vi "RT Main.vi"() -> ()   [LabVIEW 2013]
doc: "This template is for the Queued Message Handler design pattern.\n\nThe Event Handling Loop generates messages based on user interface actions.\n\nThe Message Handling Loop processes messages generated by the Event Handling Loop, or by other messages. The messages are string values, so new messages can be added easily to the Message Cases case structure in the Message Handling Loop. Each message cluster can also provide an optional value for Message Data, which is a variant that can be converted to whatever message-specific data is required."
uses:
  controls/Custom Controller Inputs.ctl
  <vilib>/userdefined/High Color/nirio_resource_hc.ctl
  controls/FPGA State.ctl
  controls/Raw Values.ctl
  controls/Control Configuration.ctl
  Globals/Global - All RT Loop Stop.vi
  Globals/Global - Configuration Options.vi
  <vilib>/rvi/errors/niLvFpgaAdjustHostInterfaceError.vi
  Globals/Global - RT Stream Connections.vi
  <vilib>/FPGAPlugInAG/cRIO-9075/niLvFpga_Close_cRIO-9075.vi
  <vilib>/rvi/interface/nirviReadWriteControl/nirviReadWriteControl.xnode
  controls/FPGA VI Reference.ctl
  FPGA Bitfiles/crio-FPGA-contro_FPGATarget_FPGAMain_4HKUk4gb9wY.lvbitx
  <vilib>/rvi/interface/nirviCloseFPGA/nirviCloseFPGA.xnode
  support/Message Queue/Message Queue.lvlib
  NiFpgaLv.dll
  <vilib>/nisyscfg/nisyscfg.lvlib
panel:
  in  "resource name":T1
  in  "Custom Controller Inputs":T2
  out "Data":T3 {"Other Controller Gains"."Position Control Kp" format="%.11g"; "Other Controller Gains"."Virtual Spring Constant (N/m)" format="%.8g"; "Other Controller Gains"."Offset weight (N)" format="%.11g"; "Other Controller Gains"."Fthresh (N)" format="%.13g"; "Other Controller Gains"."Var2" format="%.13g"}
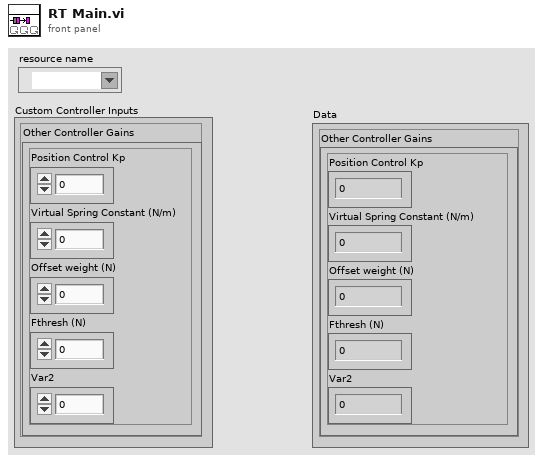
[diagram p1: front panel]
types:
  T1 = typedef "nirio_resource_hc.ctl" = tag
  T2 = typedef "Custom Controller Inputs.ctl" = cluster{"Other Controller Gains":cluster{"Position Control Kp":fxp<+/-,16,8>, "Virtual Spring Constant (N/m)":fxp<+,16,12>, "Offset weight (N)":fxp<+/-,16,8>, "Fthresh (N)":fxp<+/-,16,5>, "Var2":fxp<+/-,16,5>}}
  T3 = cluster{"Other Controller Gains":cluster{"Position Control Kp":fxp<+/-,16,8>, "Virtual Spring Constant (N/m)":fxp<+,16,12>, "Offset weight (N)":fxp<+/-,16,8>, "Fthresh (N)":fxp<+/-,16,5>, "Var2":fxp<+/-,16,5>}}
  T4 = typedef "FPGA VI Reference.ctl" = refnum<k20>
  T5 = typedef "FPGA State.ctl" = enum16{"Safe State", "Manual", "Control (PID)"}
  T6 = typedef "Raw Values.ctl" = cluster{"Channel 0":fxp<+/-,20,7>, "Channel 1":fxp<+/-,20,7>, "Channel 2":fxp<+/-,20,7>, "Channel 3":fxp<+/-,20,14>}
  T7 = typedef "Control Configuration.ctl" = cluster{"PID Gains":cluster{"proportional gain (Kc)":fxp<+/-,16,8>, "integral gain (Kc*Ts/Ti)":fxp<+/-,16,8>, "derivative gain (Kc*Td/Ts)":fxp<+/-,16,8>}, "Output Range":cluster{"output high":fxp<+/-,16,7>, "output low":fxp<+/-,16,7>}}
  T8 = typedef "All FPGA Configuration Values.ctl" = cluster{"FPGA State":T5, "Manual Values":T6, "Setpoints":T6, "Control Configurations":T7[]}
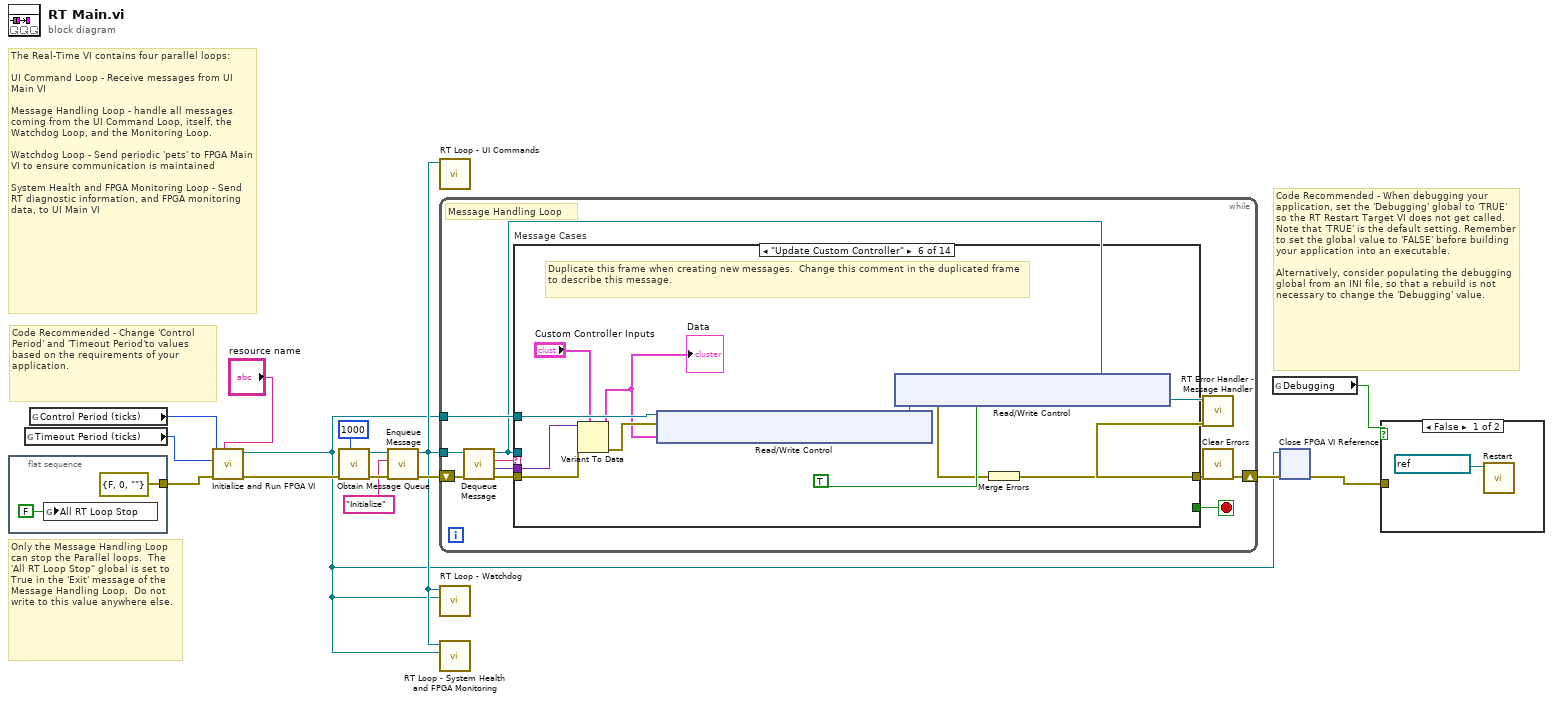
[diagram p0: block diagram]
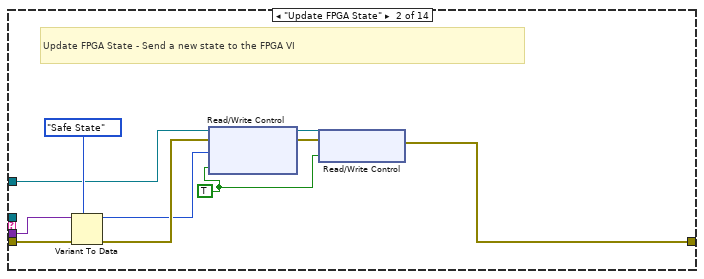
[diagram p4: hidden frame]
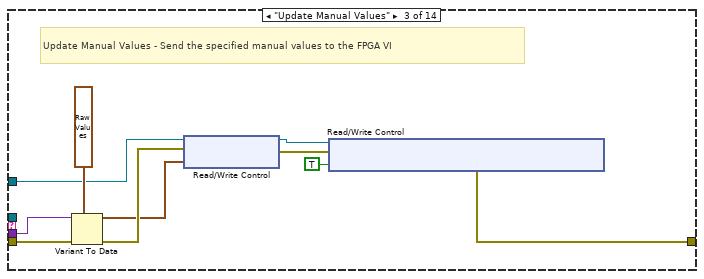
[diagram p5: hidden frame]
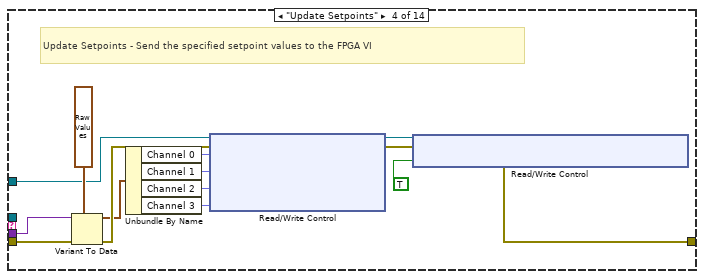
[diagram p6: hidden frame]
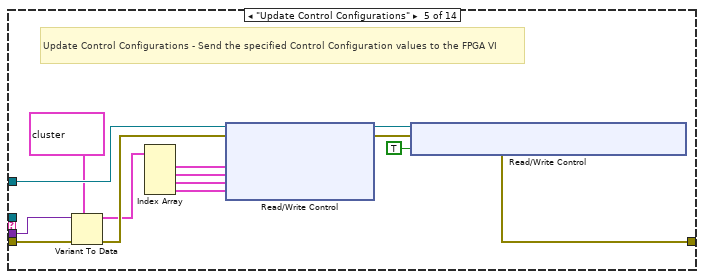
[diagram p7: hidden frame]
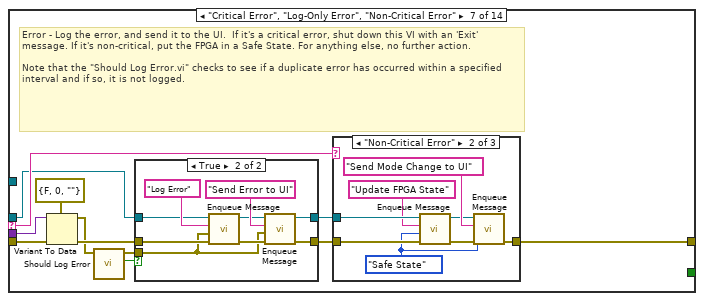
[diagram p8: hidden frame]
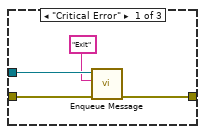
[diagram p10: hidden frame]
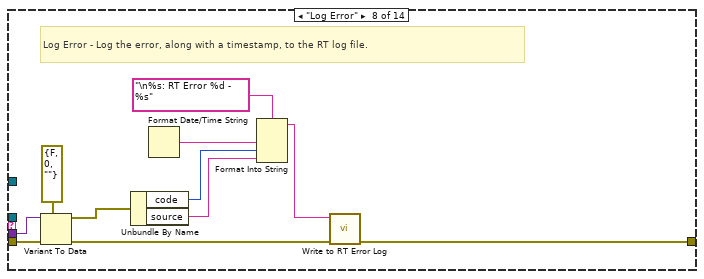
[diagram p12: hidden frame]
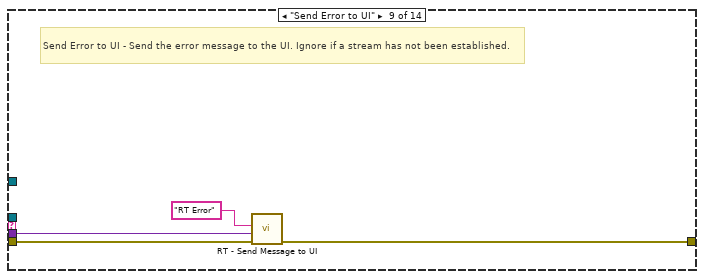
[diagram p13: hidden frame]
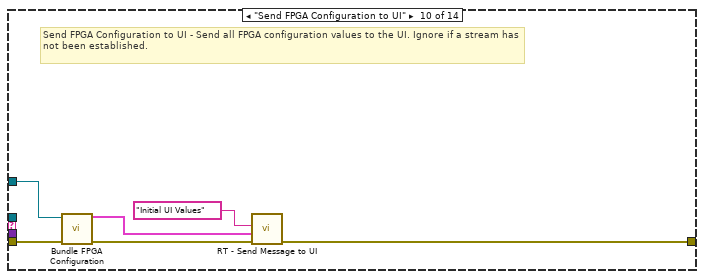
[diagram p14: hidden frame]
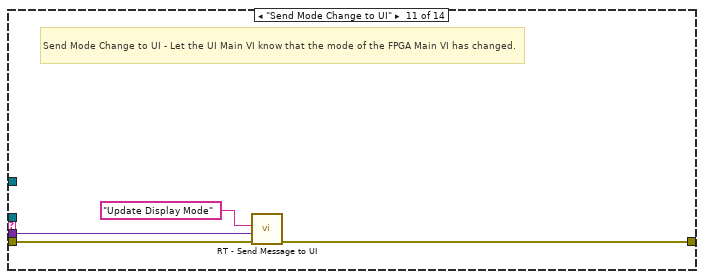
[diagram p15: hidden frame]
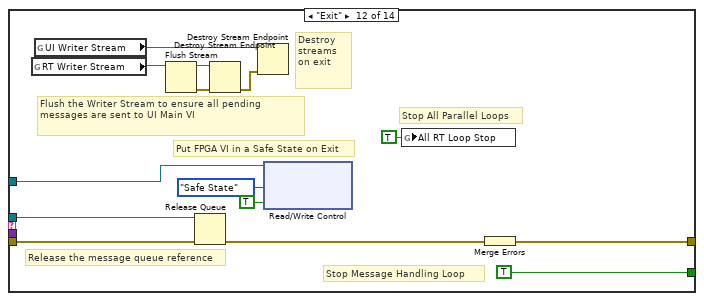
[diagram p16: hidden frame]
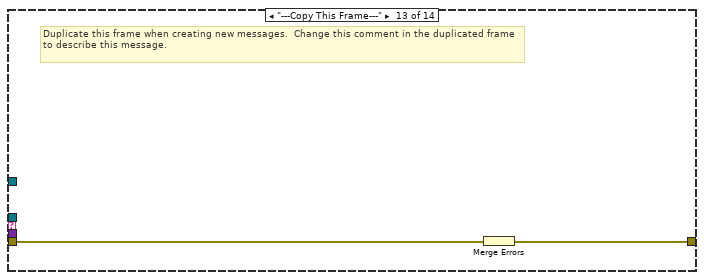
[diagram p17: hidden frame]
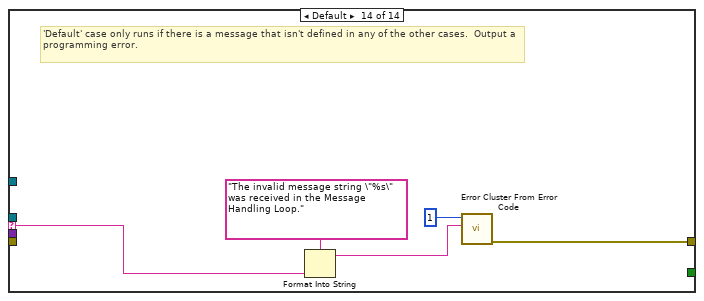
[diagram p18: hidden frame]
diagram:
  # "Code Recommended - When debugging your application, set the 'Debugging' global to 'TRUE' so the RT Restart Target VI does not get called.  Note that 'TRUE' is the default setting. Remember to set the global value to 'FALSE' before building your application into an executable.\n\nAlternatively, consider populating the debugging global from an INI file, so that a rebuild is not necessary to change the 'Debugging' value."
  # "Code Recommended - Change 'Control Period' and 'Timeout Period'to values based on the requirements of your application."
  # "The Real-Time VI contains four parallel loops:\n\nUI Command Loop - Receive messages from UI Main VI\n\nMessage Handling Loop - handle all messages coming from the UI Command Loop, itself, the Watchdog Loop, and the Monitoring Loop.\n\nWatchdog Loop - Send periodic 'pets' to FPGA Main VI to ensure communication is maintained\n\nSystem Health and FPGA Monitoring Loop - Send RT diagnostic information, and FPGA monitoring data, to UI Main VI"
  # "Only the Message Handling Loop can stop the Parallel loops.  The 'All RT Loop Stop\" global is set to True in the 'Exit' message of the Message Handling Loop.  Do not write to this value anywhere else."
  n1 = flat-sequence {
    tunnel: [errorcluster {"status"=FALSE, "code"=0, "source"=""} ("error constant")] -> w5
    frame #0 {
      n2 = global write "Global - All RT Loop Stop.vi" "All RT Loop Stop"(FALSE) -> ()
    }
  }
  n3 = global read "Global - Configuration Options.vi" "Timeout Period (ticks)"() -> (w3:u64)
  n4 = global read "Global - Configuration Options.vi" "Control Period (ticks)"() -> (w4:u32)
  n5 = call "Initialize and Run FPGA VI.vi"("resource name"="resource name", "error in (no error)"=w5, "Timeout Period (ticks)"=w3, "Control Period (ticks)"=w4) -> ("error out"=w6:errorcluster, "FPGA VI Reference Out"=w2:T4)  [unwired: 6 in]
  n6 = call "Obtain Message Queue.vi"("max queue size (-1, unlimited)"=1000, "error in (no error)"=w6) -> ("error out"=w15:errorcluster, "Message Queue"=w14:refnum<queue>)  [unwired: 8 in]
  n7 = call "Enqueue Message.vi"("error in (no error)"=w15, "Message"="Initialize", "Message Queue"=w14) -> ("error out"=w12:errorcluster, "dup Message Queue"=w11:refnum<queue>)  [unwired: 7 in]
  n8 = call "RT Loop - UI Commands.vi"("Message Queue"=w11) -> ()  [unwired: 11 in]
  n9 = while {
    tunnel: w11 -> [w22]
    shift-right: [w19] -> w10
    shift-left: w12 -> [w26]
    tunnel: w2 -> [w21]
    stop <- w27 stop-if-true
    # "Message Handling Loop"
    n10 = call "Dequeue Message.vi"("error in (no error)"=w26, "Message Queue"=w22) -> ("error out"=w25:errorcluster, "Message Data"=w23:variant, "Message"=w24:string, "dup Message Queue"=w20:refnum<queue>)  [unwired: 6 in]
    n11 = case "Message Cases" shown="\"Update Custom Controller\"" w24 {
      selector: w24 -> [_ _ _ _ _ _ w97 _ _ _ _ _ _ w168]
      tunnel: w20 -> [_ _ _ _ _ _ w91 _ _ _ _ w162 _ _]
      tunnel: w25 -> [w28 w38 w48 w62 w76 w86 w95 w134 w138 w144 w148 w158 w164 _]
      tunnel: [w28 w30 w39 w49 w63 w87 w96 w125 w135 w139 w147 w159 w163 w166] -> w18
      tunnel: [_ _ _ _ _ _ _ _ _ _ _ TRUE _ _] -> w27
      tunnel: w23 -> [_ w37 w47 w61 w75 w85 w94 w133 w137 _ w146 _ _ _]
      tunnel: w21 -> [_ w34 w44 w58 w73 w84 _ _ _ w143 _ w154 _ _]
      frame "Initialize" {
        # "Initialize - Currently a no-op for the RT Main VI"
      }
      frame "Update FPGA State" {
        w29 = TRUE ("Change State")
        # "Update FPGA State - Send a new state to the FPGA VI"
        n12 = Variant To Data(error in=w38, type=FPGA_State."Safe State" ("FPGA State"), Variant=w37) -> (data=w33:T5, error out=w35:errorcluster)
        n13 = xnode "Read/Write Control"("FPGA VI Reference In"=w34, "error in"=w35, "New State"=w33, "Change State"=w29) -> ("FPGA VI Reference Out"=w32:T4, "error out"=w31:errorcluster)
        n14 = xnode "Read/Write Control"("FPGA VI Reference In"=w32, "error in"=w31, "Disable Drive"=w29) -> ("error out"=w30:errorcluster)  [unwired: 1 out]
      }
      frame "Update Manual Values" {
        # "Update Manual Values - Send the specified manual values to the FPGA VI"
        n15 = Variant To Data(error in=w48, type=T6 {"Channel 0"=0.0, "Channel 1"=0.0, "Channel 2"=0.0, "Channel 3"=0.0} ("Raw Values"), Variant=w47) -> (data=w43:T6, error out=w45:errorcluster)
        n16 = xnode "Read/Write Control"("FPGA VI Reference In"=w44, "error in"=w45, "Manual Values"=w43) -> ("FPGA VI Reference Out"=w42:T4, "error out"=w41:errorcluster)
        n17 = xnode "Read/Write Control"("FPGA VI Reference In"=w42, "error in"=w41, "Enable Drive"=TRUE) -> ("error out"=w39:errorcluster)  [unwired: 1 out]
      }
      frame "Update Setpoints" {
        # "Update Setpoints - Send the specified setpoint values to the FPGA VI"
        n18 = Variant To Data(error in=w62, type=T6 {"Channel 0"=0.0, "Channel 1"=0.0, "Channel 2"=0.0, "Channel 3"=0.0} ("Raw Values"), Variant=w61) -> (data=w57:T6, error out=w59:errorcluster)
        n19 = Unbundle By Name(w57) -> ("Channel 0"=w56:fxp<+/-,20,7>, "Channel 1"=w53:fxp<+/-,20,7>, "Channel 2"=w55:fxp<+/-,20,7>, "Channel 3"=w54:fxp<+/-,20,14>)
        n20 = xnode "Read/Write Control"("FPGA VI Reference In"=w58, "error in"=w59, "Channel 0 Setpoint (Force)"=w56, "Channel 1 Setpoint  (Position)"=w53, "Channel 2 Setpoint"=w55, "Channel 3 Setpoint"=w54) -> ("FPGA VI Reference Out"=w50:T4, "error out"=w51:errorcluster)
        n21 = xnode "Read/Write Control"("FPGA VI Reference In"=w50, "error in"=w51, "Enable Drive"=TRUE) -> ("error out"=w49:errorcluster)  [unwired: 1 out]
      }
      frame "Update Control Configurations" {
        # "Update Control Configurations - Send the specified Control Configuration values to the FPGA VI"
        n22 = Variant To Data(error in=w76, type=T7[] [{"PID Gains"={"proportional gain (Kc)"=0.0, "integral gain (Kc*Ts/Ti)"=0.0, "derivative gain (Kc*Td/Ts)"=0.0}, "Output Range"={"output high"=0.0, "output low"=0.0}}], Variant=w75) -> (data=w71:T7[], error out=w74:errorcluster)
        n23 = Index Array(array=w71) -> (element #1=w70:T7, element #2=w69:T7, element #3=w68:T7, element #4=w67:T7)  [unwired: 4 in]
        n24 = xnode "Read/Write Control"("FPGA VI Reference In"=w73, "error in"=w74, "Channel 0 Configuration"=w70, "Channel 1 Configuration"=w69, "Channel 2 Configuration"=w68, "Channel 3 Configuration"=w67) -> ("FPGA VI Reference Out"=w65:T4, "error out"=w64:errorcluster)
        n25 = xnode "Read/Write Control"("FPGA VI Reference In"=w65, "error in"=w64, "Enable Drive"=TRUE) -> ("error out"=w63:errorcluster)  [unwired: 1 out]
      }
      frame "Update Custom Controller" {
        # "Duplicate this frame when creating new messages.  Change this comment in the duplicated frame to describe this message."
        n26 = Variant To Data(error in=w86, type="Custom Controller Inputs", Variant=w85) -> (data=w78:T2, error out=w83:errorcluster)
        "Data" <- w78
        n27 = xnode "Read/Write Control"("FPGA VI Reference In"=w84, "error in"=w83, "Custom Controller Inputs"=w78) -> ("FPGA VI Reference Out"=w81:T4, "error out"=w80:errorcluster)
        n28 = xnode "Read/Write Control"("FPGA VI Reference In"=w81, "error in"=w80, "Enable Drive"=TRUE) -> ("error out"=w79:errorcluster)  [unwired: 1 out]
        n29 = Merge Errors(w79) -> (w87:errorcluster)
      }
      frame "Critical Error", "Log-Only Error", "Non-Critical Error" {
        # "Error - Log the error, and send it to the UI.  If it's a critical error, shut down this VI with an 'Exit' message. If it's non-critical, put the FPGA in a Safe State. For anything else, no further action.\n\nNote that the \"Should Log Error.vi\" checks to see if a duplicate error has occurred within a specified interval and if so, it is not logged."
        n30 = Variant To Data(error in=w95, type=errorcluster {"status"=FALSE, "code"=0, "source"=""} ("error out"), Variant=w94) -> (data=w89:errorcluster, error out=w92:errorcluster)
        n31 = call "Should Log Error.vi"("error to report"=w89) -> ("Should Log Error?"=w90:bool, "dup error to report"=w88:errorcluster)  [unwired: 9 in]
        n32 = case shown="True" w90 {
          tunnel: [w101 w108] -> w99
          tunnel: [w100 w107] -> w98
          tunnel: w91 -> [w100 w106]
          tunnel: w92 -> [w101 w103]
          tunnel: w88 -> [_ w102]
          frame False {
          }
          frame True {
            n33 = call "Enqueue Message.vi"("error in (no error)"=w103, "Message Data"=w102, "Message"="Log Error", "Message Queue"=w106) -> ("error out"=w104:errorcluster, "dup Message Queue"=w105:refnum<queue>)  [unwired: 6 in]
            n34 = call "Enqueue Message.vi"("error in (no error)"=w104, "Message Data"=w102, "Message"="Send Error to UI", "Message Queue"=w105) -> ("error out"=w108:errorcluster, "dup Message Queue"=w107:refnum<queue>)  [unwired: 6 in]
          }
        }
        n35 = case shown="\"Non-Critical Error\"" w97 {
          tunnel: w99 -> [w114 w122 w123]
          tunnel: w98 -> [w112 w121 _]
          tunnel: [w113 w118 w123] -> w96
          frame "Critical Error" {
            n36 = call "Enqueue Message.vi"("error in (no error)"=w114, "Message"="Exit", "Message Queue"=w112) -> ("error out"=w113:errorcluster)  [unwired: 7 in, 1 out]
          }
          frame "Non-Critical Error" {
            w115 = FPGA_State."Safe State" ("FPGA State")
            n37 = call "Enqueue Message.vi"("error in (no error)"=w122, "Message Data"=w115, "Message"="Update FPGA State", "Message Queue"=w121) -> ("error out"=w119:errorcluster, "dup Message Queue"=w116:refnum<queue>)  [unwired: 6 in]
            n38 = call "Enqueue Message.vi"("error in (no error)"=w119, "Message Data"=w115, "Message"="Send Mode Change to UI", "Message Queue"=w116) -> ("error out"=w118:errorcluster)  [unwired: 6 in, 1 out]
          }
          frame Default {
          }
        }
      }
      frame "Log Error" {
        # "Log Error - Log the error, along with a timestamp, to the RT log file."
        n39 = Variant To Data(error in=w134, type=errorcluster {"status"=FALSE, "code"=0, "source"=""} ("error constant"), Variant=w133) -> (data=w128:errorcluster, error out=w131:errorcluster)
        n40 = Unbundle By Name(w128) -> ("code"=w127:i32, "source"=w126:string)
        n41 = Format Date/Time String() -> (date/time string=w129:string)  [unwired: 3 in]
        n42 = Format Into String(format string="\n%s: RT Error %d - %s", w129, w127, w126) -> (resulting string=w124:string)  [unwired: 2 in, 1 out]
        n43 = call "Write to RT Error Log.vi"("error in (no error)"=w131, "Log Entry"=w124) -> ("error out"=w125:errorcluster)  [unwired: 9 in]
      }
      frame "Send Error to UI" {
        # "Send Error to UI - Send the error message to the UI. Ignore if a stream has not been established."
        n44 = call "RT - Send Message to UI.vi"("error in (no error)"=w138, "Message Data"=w137, "Message"="RT Error") -> ("error out"=w135:errorcluster)  [unwired: 8 in]
      }
      frame "Send FPGA Configuration to UI" {
        # "Send FPGA Configuration to UI - Send all FPGA configuration values to the UI. Ignore if a stream has not been established."
        n45 = call "Bundle FPGA Configuration.vi"("error in (no error)"=w144, "FPGA Interface (Old)"=w143) -> ("error out"=w142:errorcluster, "All FPGA Configuration Values"=w141:T8)  [unwired: 8 in]
        n46 = call "RT - Send Message to UI.vi"("error in (no error)"=w142, "Message Data"=w141, "Message"="Initial UI Values") -> ("error out"=w139:errorcluster)  [unwired: 8 in]
      }
      frame "Send Mode Change to UI" {
        # "Send Mode Change to UI - Let the UI Main VI know that the mode of the FPGA Main VI has changed."
        n47 = call "RT - Send Message to UI.vi"("error in (no error)"=w148, "Message Data"=w146, "Message"="Update Display Mode") -> ("error out"=w147:errorcluster)  [unwired: 8 in]
      }
      frame "Exit" {
        # "Flush the Writer Stream to ensure all pending messages are sent to UI Main VI"
        # "Destroy streams on exit"
        # "Put FPGA VI in a Safe State on Exit"
        # "Stop Message Handling Loop"
        # "Stop All Parallel Loops"
        # "Release the message queue reference"
        n48 = global read "Global - RT Stream Connections.vi" "RT Writer Stream"() -> (w151:refnum<k21>)
        n49 = global read "Global - RT Stream Connections.vi" "UI Writer Stream"() -> (w153:refnum<k21>)
        n50 = Flush Stream(11:w151) -> (0:w149:errorcluster, 3:w150:refnum<k21>)  [unwired: 3 in, 1 out]
        n51 = Release Queue(queue=w162, error in (no error)=w158) -> (error out=w160:errorcluster)  [unwired: 1 in, 2 out]
        n52 = Destroy Stream Endpoint(8:w149, 11:w150) -> (0:w152:errorcluster)
        n53 = Destroy Stream Endpoint(8:w152, 11:w153) -> ()  [unwired: 1 out]
        n54 = xnode "Read/Write Control"("FPGA VI Reference In"=w154, "New State"=FPGA_State."Safe State", "Change State"=TRUE) -> ()  [unwired: 1 in, 2 out]
        n55 = global write "Global - All RT Loop Stop.vi" "All RT Loop Stop"(TRUE ("Stop Monitoring Loops")) -> ()
        n56 = Merge Errors(w160) -> (w159:errorcluster)
      }
      frame "---Copy This Frame---" {
        # "Duplicate this frame when creating new messages.  Change this comment in the duplicated frame to describe this message."
        n57 = Merge Errors(w164) -> (w163:errorcluster)
      }
      frame Default {
        # "'Default' case only runs if there is a message that isn't defined in any of the other cases.  Output a programming error."
        n58 = Format Into String(format string="The invalid message string \"%s\" was received in the Message Handling Loop." ("Unknown Message Error Text"), w168) -> (resulting string=w165:string)  [unwired: 2 in, 1 out]
        n59 = call <vilib>:"Error Cluster From Error Code.vi"("error message (\"\")"=w165, "error code (0)"=1) -> ("error out"=w166:errorcluster)  [unwired: 7 in]
      }
    }
    n60 = call "RT Error Handler - Message Handler.vi"("error in (no error)"=w18, "Message Queue"=w20) -> ()  [unwired: 9 in, 1 out]
    n61 = call <vilib>:"Clear Errors.vi"("error in (no error)"=w18) -> ("error out"=w19:errorcluster)  [unwired: 6 in]
  }
  n62 = call "RT Loop - Watchdog.vi"("FPGA VI Reference(Old)"=w2, "Message Queue"=w11) -> ()  [unwired: 10 in]
  n63 = call "RT Loop - System Health and FPGA Monitoring.vi"("FPGA VI Reference (Old)"=w2, "Message Queue"=w11) -> ()  [unwired: 10 in]
  n64 = global read "Global - Configuration Options.vi" "Debugging"() -> (w8:bool)
  n65 = xnode "Close FPGA VI Reference"("FPGA VI Reference In"=w2, "error in"=w10) -> ("error out"=w9:errorcluster)
  n66 = case shown="False" w8 {
    tunnel: w9 -> [_ _]
    frame False {
      n67 = call <vilib>:"Restart.vi"("session in"=refnum<k21> "localhost") -> ()  [unwired: 8 in, 3 out]
    }
    frame True {
    }
  }
